vi "Tree.vi"   [LabVIEW 2016, in "LockinDAQ.lvclass"]
uses:
  LockinDAQ.lvclass
  Instrument.Lockin/Instrument.Lockin.lvclass
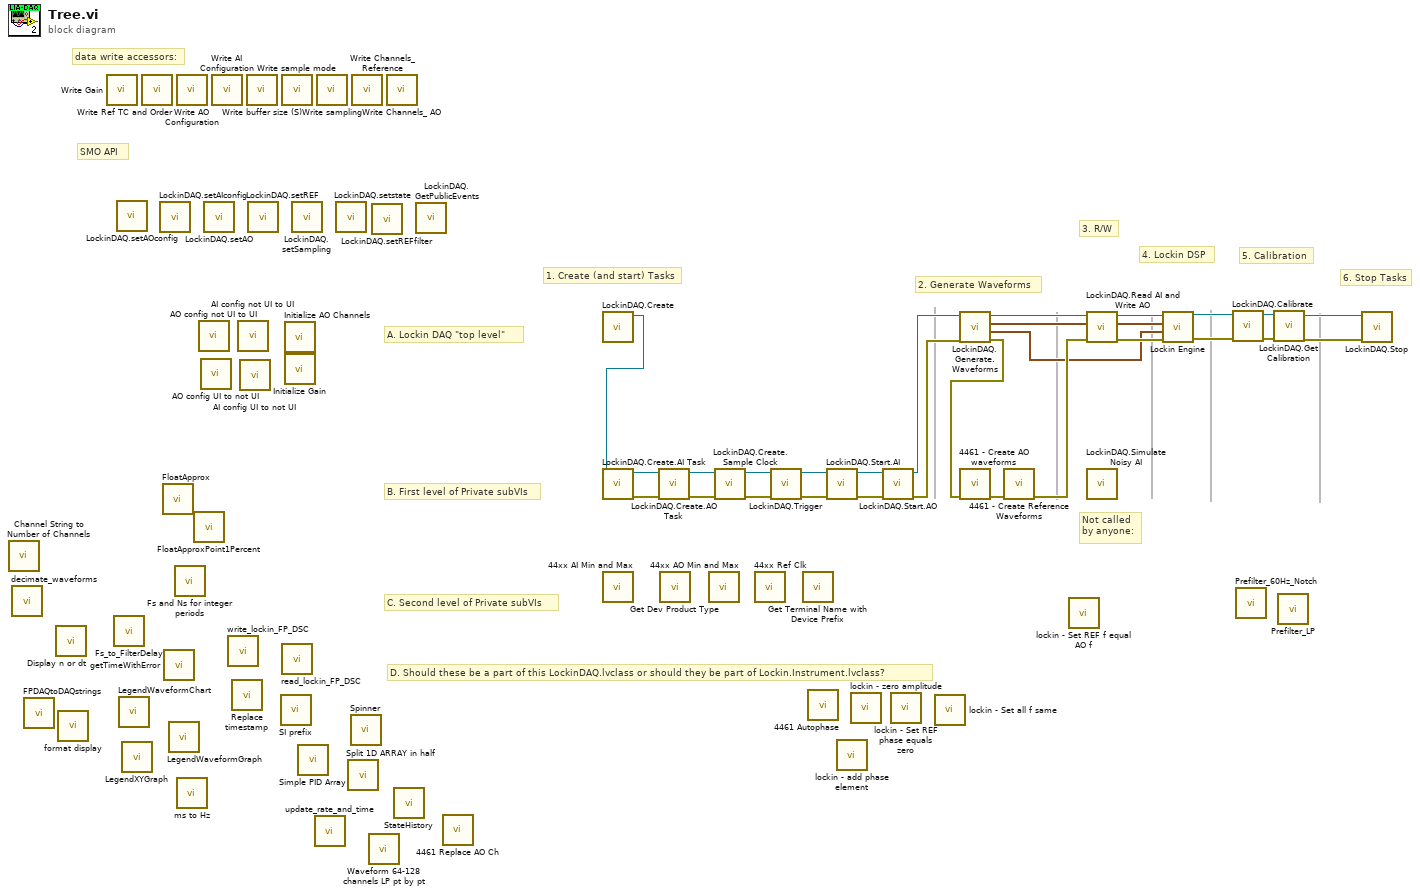
[diagram p0: block diagram]
diagram:
  # "SMO API"
  # "data write accessors:"
  # "D. Should these be a part of this LockinDAQ.lvclass or should they be part of Lockin.Instrument.lvclass?"
  # "B. First level of Private subVIs"
  # "6. Stop Tasks"
  # "5. Calibration"
  # "4. Lockin DSP"
  # "3. R/W"
  # "2. Generate Waveforms"
  # "A. Lockin DAQ \"top level\""
  # "1. Create (and start) Tasks"
  # "Not called\nby anyone:"
  # "C. Second level of Private subVIs"
  n1 = call "Channel String to Number of Channels.vi"() -> ()  [unwired: 5 in, 1 out]
  n2 = call "decimate_waveforms.vi"() -> ()  [unwired: 9 in, 2 out]
  n3 = call "FPDAQtoDAQstrings.vi"() -> ()  [unwired: 1 in, 1 out]
  n4 = call "Display n or dt.vi"() -> ()  [unwired: 10 in, 2 out]
  n5 = call "format display.vi"() -> ()  [unwired: 6 in, 6 out]
  n6 = call "Write Gain.vi"() -> ()  [unwired: 10 in, 2 out]
  n7 = call "Fs_to_FilterDelay.vi"() -> ()  [unwired: 11 in, 1 out]
  n8 = call "LockinDAQ.setAOconfig.vi"() -> ()  [unwired: 10 in, 2 out]
  n9 = call "LegendWaveformChart.vi"() -> ()  [unwired: 9 in, 3 out]
  n10 = call "LegendXYGraph.vi"() -> ()  [unwired: 9 in, 3 out]
  n11 = call "Write Ref TC and Order.vi"() -> ()  [unwired: 10 in, 2 out]
  n12 = call "LockinDAQ.setAIconfig.vi"() -> ()  [unwired: 10 in, 2 out]
  n13 = call "FloatApprox.vi"() -> ()  [unwired: 4 in, 1 out]
  n14 = call "getTimeWithError.vi"() -> ()  [unwired: 10 in, 2 out]
  n15 = call "LegendWaveformGraph.vi"() -> ()  [unwired: 9 in, 3 out]
  n16 = call "Fs and Ns for integer periods.vi"() -> ()  [unwired: 10 in, 2 out]
  n17 = call "Write AO Configuration.vi"() -> ()  [unwired: 10 in, 2 out]
  n18 = call "ms to Hz.vi"() -> ()  [unwired: 1 in, 1 out]
  n19 = call "FloatApproxPoint1Percent.vi"() -> ()  [unwired: 4 in, 1 out]
  n20 = call "AO config not UI to UI.vi"() -> ()  [unwired: 10 in, 2 out]
  n21 = call "AO config UI to not UI.vi"() -> ()  [unwired: 11 in, 1 out]
  n22 = call "LockinDAQ.setAO.vi"() -> ()  [unwired: 10 in, 2 out]
  n23 = call "Write AI Configuration.vi"() -> ()  [unwired: 10 in, 2 out]
  n24 = call "write_lockin_FP_DSC.vi"() -> ()  [unwired: 11 in, 1 out]
  n25 = call "Replace timestamp.vi"() -> ()  [unwired: 11 in, 1 out]
  n26 = call "AI config not UI to UI.vi"() -> ()  [unwired: 9 in, 3 out]
  n27 = call "AI config UI to not UI.vi"() -> ()  [unwired: 11 in, 1 out]
  n28 = call "Write buffer size (S).vi"() -> ()  [unwired: 10 in, 2 out]
  n29 = call "LockinDAQ.setREF.vi"() -> ()  [unwired: 10 in, 2 out]
  n30 = call "SI prefix.vi"() -> ()  [unwired: 1 in, 1 out]
  n31 = call "Write sample mode.vi"() -> ()  [unwired: 10 in, 2 out]
  n32 = call "read_lockin_FP_DSC.vi"() -> ()  [unwired: 10 in, 2 out]
  n33 = call "Initialize AO Channels.vi"() -> ()  [unwired: 9 in, 3 out]
  n34 = call "Initialize Gain.vi"() -> ()  [unwired: 9 in, 3 out]
  n35 = call "LockinDAQ.setSampling.vi"() -> ()  [unwired: 10 in, 2 out]
  n36 = call "Simple PID Array.vi"() -> ()  [unwired: 11 in, 1 out]
  n37 = call "update_rate_and_time.vi"() -> ()  [unwired: 9 in, 3 out]
  n38 = call "Write sampling.vi"() -> ()  [unwired: 10 in, 2 out]
  n39 = call "LockinDAQ.setstate.vi"() -> ()  [unwired: 10 in, 2 out]
  n40 = call "Split 1D ARRAY in half.vi"() -> ()  [unwired: 9 in, 3 out]
  n41 = call "Spinner.vi"() -> ()  [unwired: 5 in, 1 out]
  n42 = call "Write Channels_ Reference.vi"() -> ()  [unwired: 10 in, 2 out]
  n43 = call "Waveform 64-128 channels LP pt by pt.vi"() -> ()  [unwired: 11 in, 1 out]
  n44 = call "LockinDAQ.setREFfilter.vi"() -> ()  [unwired: 10 in, 2 out]
  n45 = call "Write Channels_ AO.vi"() -> ()  [unwired: 10 in, 2 out]
  n46 = call "StateHistory.vi"() -> ()  [unwired: 9 in, 2 out]
  n47 = call "LockinDAQ.GetPublicEvents.vi"() -> ()  [unwired: 9 in, 3 out]
  n48 = call "4461 Replace AO Ch.vi"() -> ()  [unwired: 10 in, 2 out]
  n49 = call "LockinDAQ.Create.vi"() -> ("LockinDAQ out"=w20:refnum<class "LockinDAQ.lvclass">)  [unwired: 10 in, 1 out]
  n50 = call "LockinDAQ.Create.AI Task.vi"("LockinDAQ"=w20) -> ("error out"=w18:errorcluster, "LockinDAQ out"=w19:refnum<class "LockinDAQ.lvclass">)  [unwired: 9 in]
  n51 = call "44xx AI Min and Max.vi"() -> ()  [unwired: 9 in, 3 out]
  n52 = call "LockinDAQ.Create.AO Task.vi"("error in (no error)"=w18, "LockinDAQ"=w19) -> ("error out"=w16:errorcluster, "LockinDAQ out"=w17:refnum<class "LockinDAQ.lvclass">)  [unwired: 8 in]
  n53 = call "Get Dev Product Type.vi"() -> ()  [unwired: 8 in, 4 out]
  n54 = call "44xx AO Min and Max.vi"() -> ()  [unwired: 9 in, 3 out]
  n55 = call "LockinDAQ.Create.Sample Clock.vi"("error in (no error)"=w16, "LockinDAQ"=w17) -> ("error out"=w14:errorcluster, "LockinDAQ out"=w15:refnum<class "LockinDAQ.lvclass">)  [unwired: 8 in]
  n56 = call "44xx Ref Clk.vi"() -> ()  [unwired: 9 in, 3 out]
  n57 = call "LockinDAQ.Trigger.vi"("error in (no error)"=w14, "LockinDAQ"=w15) -> ("error out"=w12:errorcluster, "LockinDAQ out"=w13:refnum<class "LockinDAQ.lvclass">)  [unwired: 8 in]
  n58 = call "Get Terminal Name with Device Prefix.vi"() -> ()  [unwired: 9 in, 3 out]
  n59 = call "4461 Autophase.vi"() -> ()  [unwired: 10 in, 2 out]
  n60 = call "LockinDAQ.Start.AI.vi"("error in (no error)"=w12, "LockinDAQ"=w13) -> ("error out"=w10:errorcluster, "LockinDAQ out"=w11:refnum<class "LockinDAQ.lvclass">)  [unwired: 6 in]
  n61 = call "lockin - add phase element.vi"() -> ()  [unwired: 10 in, 2 out]
  n62 = call "lockin - zero amplitude.vi"() -> ()  [unwired: 10 in, 2 out]
  n63 = call "LockinDAQ.Start.AO.vi"("error in (no error)"=w10, "LockinDAQ"=w11) -> ("error out"=w4:errorcluster, "LockinDAQ out"=w9:refnum<class "LockinDAQ.lvclass">)  [unwired: 8 in]
  n64 = call "lockin - Set REF phase equals zero.vi"() -> ()  [unwired: 10 in, 2 out]
  n65 = call "lockin - Set all f same.vi"() -> ()  [unwired: 10 in, 2 out]
  n66 = call "LockinDAQ.Generate.Waveforms.vi"("error in (no error)"=w4, "LockinDAQ"=w9) -> ("error out"=w8:errorcluster, "REF []"=w1:waveform(dbl)[], "AO []"=w2:waveform(dbl)[], "LockinDAQ out"=w5:refnum<class "LockinDAQ.lvclass">)  [unwired: 6 in]
  n67 = call "4461 - Create AO waveforms.vi"("error in (no error)"=w8) -> ("error out"=w7:errorcluster)  [unwired: 7 in, 3 out]
  n68 = call "4461 - Create Reference Waveforms.vi"("error in (no error)"=w7) -> ("error out"=w6:errorcluster)  [unwired: 7 in, 3 out]
  n69 = call "lockin - Set REF f equal AO f.vi"() -> ()  [unwired: 10 in, 2 out]
  n70 = call "LockinDAQ.Read AI and Write AO.vi"("error in (no error)"=w6, "AO []"=w2, "LockinDAQ"=w5) -> ("error out"=w27:errorcluster, "AI []"=w3:waveform(dbl)[], "LockinDAQ out"=w28:refnum<class "LockinDAQ.lvclass">)  [unwired: 6 in]
  n71 = call "LockinDAQ.Simulate Noisy AI.vi"() -> ()  [unwired: 9 in, 3 out]
  n72 = call "Lockin Engine.vi"("error in (no error)"=w27, "Reference In"=w1, "Signal in"=w3, "LockinDAQ"=w28) -> ("error out"=w25:errorcluster, "LockinDAQ out"=w26:refnum<class "LockinDAQ.lvclass">)  [unwired: 4 in, 2 out]
  n73 = call "LockinDAQ.Calibrate.vi"("error in (no error)"=w25, "LockinDAQ"=w26) -> ("error out"=w23:errorcluster, "LockinDAQ out"=w24:refnum<class "LockinDAQ.lvclass">)  [unwired: 7 in, 1 out]
  n74 = call "Prefilter_60Hz_Notch.vi"() -> ()  [unwired: 10 in, 2 out]
  n75 = call "LockinDAQ.Get Calibration.vi"("error in (no error)"=w23, "LockinDAQ"=w24) -> ("error out"=w21:errorcluster, "LockinDAQ out"=w22:refnum<class "LockinDAQ.lvclass">)  [unwired: 7 in, 1 out]
  n76 = call "Prefilter_LP.vi"() -> ()  [unwired: 10 in, 2 out]
  n77 = call "LockinDAQ.Stop.vi"("error in (no error)"=w21, "LockinDAQ"=w22) -> ()  [unwired: 8 in, 2 out]
